vi "Main.vi"() -> ()   [LabVIEW 2017, in "FingerPrintMânager.lvlib"]
doc: "This template is based off of the Queued Message Handler design pattern and the Queued Message Handler project template that ships with LabVIEW.\n\nThe main difference is that the queue is private to this module and communication between modules is performed via Broadcast and Request events.\n\nRequest events are wrapped in public API methods and are handled in the Event Handling Loop (EHL) of this VI. Any module can register for Broadcast events sent by this module. The EHL generates messages based on user interface actions.\n\nThe Message Handling Loop (MHL) processes messages generated by the EHL, or by other messages. The messages are string values, so new messages can be added easily to the Message Cases case structure in the MHL. Each message cluster can also provide an optional value for Message Data, which is a variant that can be converted to whatever message-specific data is required.\n_____\nBased on Delacor QMH Project Template 4.1.0.59."
uses:
  <vilib>/Delacor/Delacor QMH/Libraries/Module Admin_class/Delacor_lib_QMH_Module Admin.lvclass
  Module Data--cluster.ctl
  Stop Argument--cluster.ctl
  <vilib>/Delacor/Delacor QMH/Libraries/Module Admin_class/Delacor_lib_QMH_Module Admin.lvclass/Delacor_lib_QMH_Module Admin.ctl
  Init Argument--cluster.ctl
  Init (Reply Payload)--cluster.ctl
  UnInit Argument--cluster.ctl
  Write Argument--cluster.ctl
  Write (Reply Payload)--cluster.ctl
  Read Argument--cluster.ctl
  Read (Reply Payload)--cluster.ctl
  <vilib>/Utility/miscctls.llb/LVPointTypeDef.ctl
  <vilib>/Delacor/Delacor QMH/Libraries/Module Admin_class/Delacor_lib_QMH_Get External Launch.vi
  <vilib>/Utility/error.llb/Error Cluster From Error Code.vi
  <vilib>/Delacor/Delacor QMH/Libraries/Message Queue_class/Delacor_lib_QMH_Enqueue Message (Single).vi
  <vilib>/ErrorRing/Error Ring.xnode
  <vilib>/Delacor/Delacor QMH/Libraries/Message Queue_class/Delacor_lib_QMH_Message Queue.lvclass
panel:
  out "String":string
  out "VisaRef":refnum<visa-resource-name>
  out "Connected":bool
  in  "Simulate MHL Error":bool
  in  "Simulate EHL Error":bool
  out "error out":errorcluster
  in  "Module Admin":refnum<class "Delacor_lib_QMH_Module Admin.lvclass">
  out "Status":string
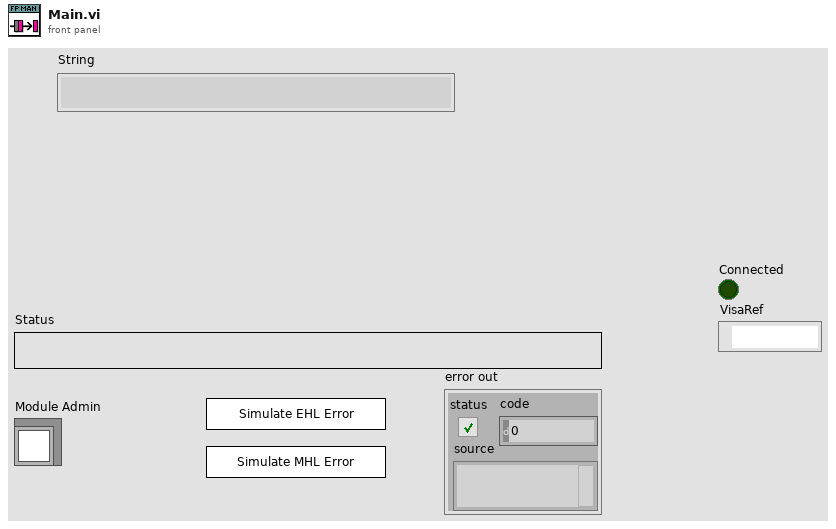
[diagram p1: front panel]
types:
  T1 = typedef "FingerPrintMânager.lvlib/Request Events--cluster.ctl" = cluster{"Stop Module":refnum<user-event>, "Show Panel":refnum<user-event>, "Hide Panel":refnum<user-event>, "Get Module Execution Status":refnum<user-event>, "Show Diagram":refnum<user-event>, "Init":refnum<user-event>, "UnInit":refnum<user-event>, "Write":refnum<user-event>, "Read":refnum<user-event>, "UpdatePump":refnum<user-event>, "StopPump":refnum<user-event>}
  T2 = typedef "FingerPrintMânager.lvlib/Module Data--cluster.ctl" = cluster{"Status":string, "VisaRef":refnum<visa-resource-name>, "Connected":bool}
  T3 = enum32{"invalid lock state", "Not Locked", "Locked (No Password)", "Password-protected"}
  T4 = typedef "FingerPrintMânager.lvlib/Stop Argument--cluster.ctl" = cluster{"Origin":string, "Exit via Stop Module Req?":bool, "Wait for Module to stop?":bool}
  T5 = typedef "FingerPrintMânager.lvlib/Init Argument--cluster.ctl" = cluster{"Wait Notifier":refnum<notifier>, "wait for reply":bool}
  T6 = typedef "FingerPrintMânager.lvlib/UnInit Argument--cluster.ctl" = cluster{"Boolean":bool}
  T7 = typedef "FingerPrintMânager.lvlib/Write Argument--cluster.ctl" = cluster{"Command":string, "Wait Notifier":refnum<notifier>, "wait for reply":bool}
  T8 = typedef "FingerPrintMânager.lvlib/Read Argument--cluster.ctl" = cluster{"Wait Notifier":refnum<notifier>, "wait for reply":bool}
  T9 = typedef "LVPointTypeDef.ctl" = cluster{"Horizontal":i16, "Vertical":i16}
  T10 = enum32{"Invalid", "Standard", "Closed", "Hidden", "Minimized", "Maximized"}
  T11 = typedef "FingerPrintMânager.lvlib/Init (Reply Payload)--cluster.ctl" = cluster{"Connected":bool, "Init_error":errorcluster}
  T12 = typedef "FingerPrintMânager.lvlib/Write (Reply Payload)--cluster.ctl" = cluster{"Status":bool, "Write_error":errorcluster}
  T13 = typedef "FingerPrintMânager.lvlib/Read (Reply Payload)--cluster.ctl" = cluster{"Status":bool, "Response":string, "Read_error":errorcluster}
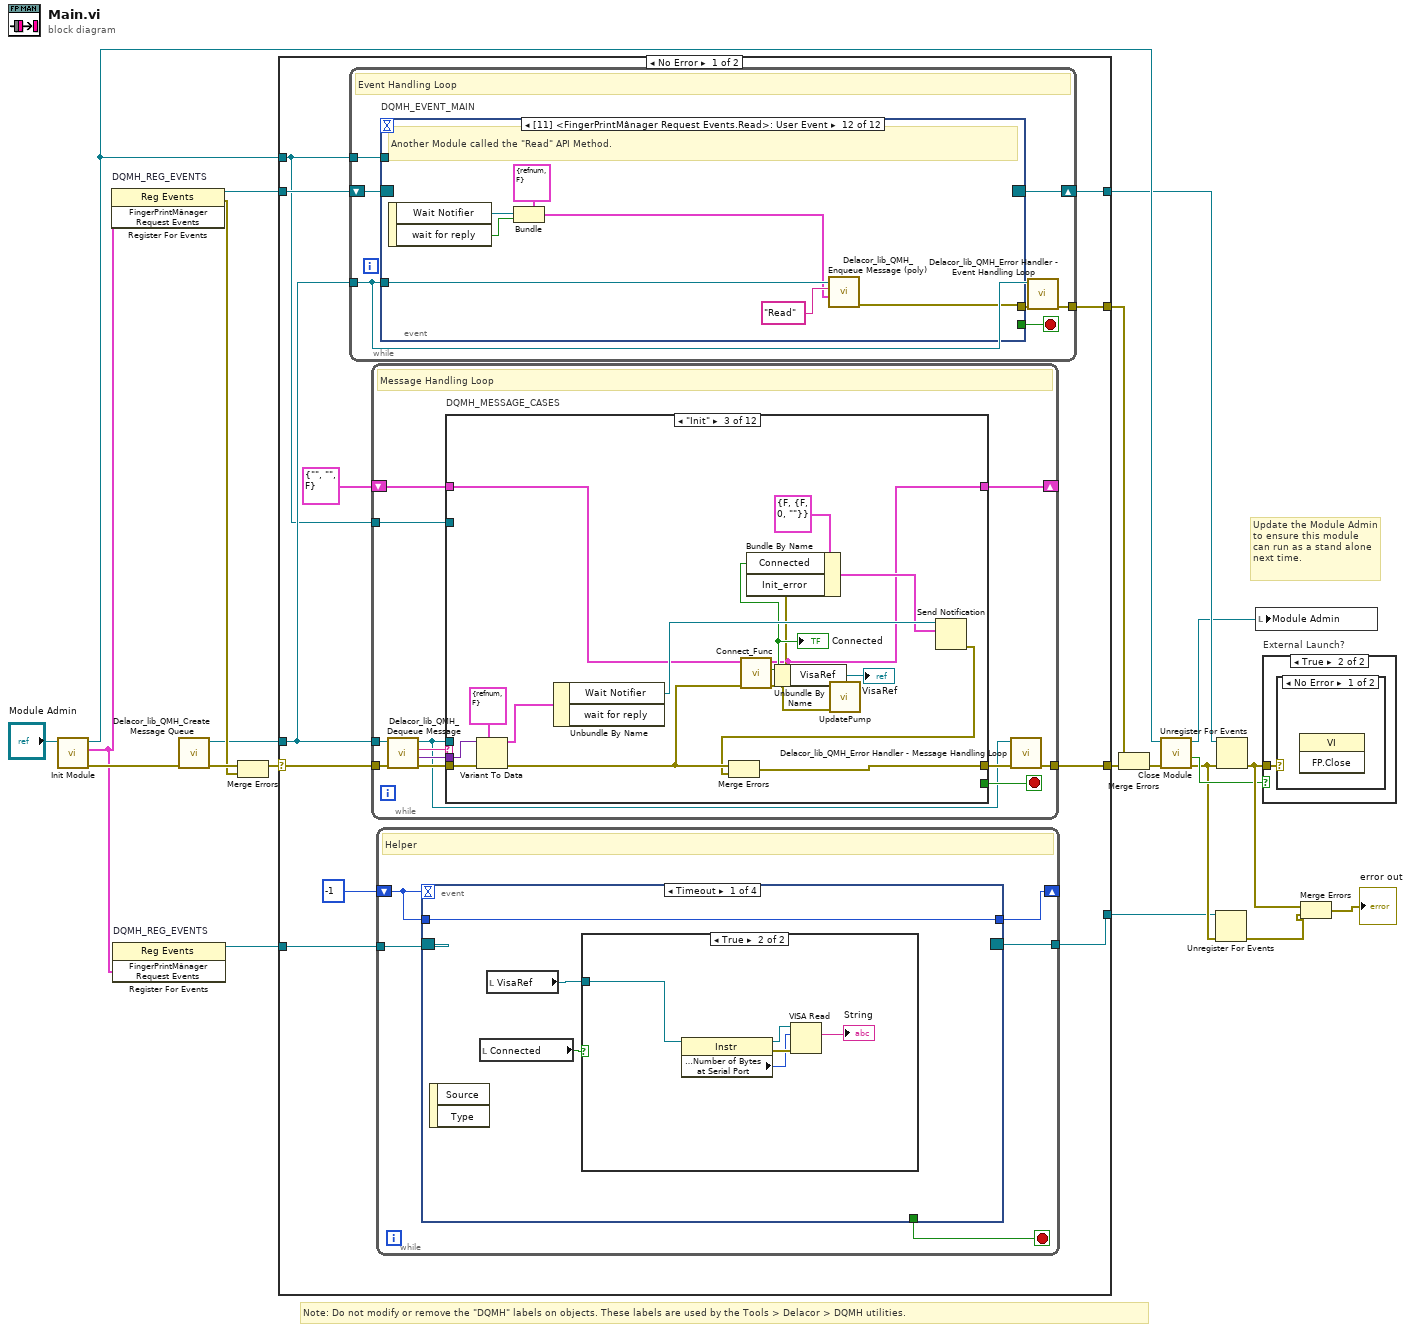
[diagram p0: block diagram]
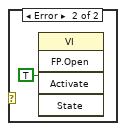
[diagram p3: hidden frame]
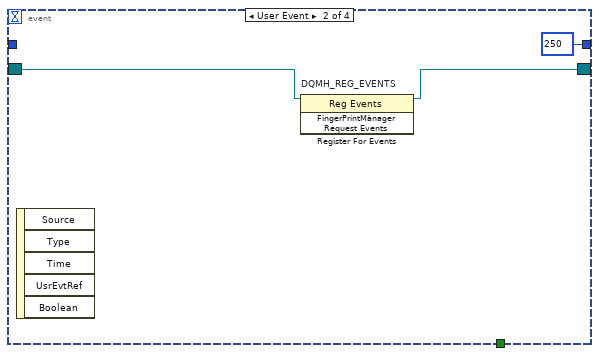
[diagram p5: hidden frame]
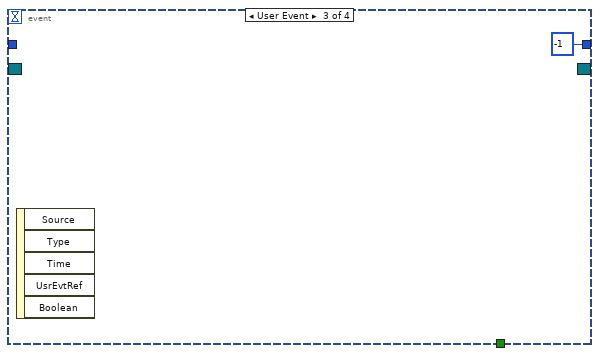
[diagram p6: hidden frame]
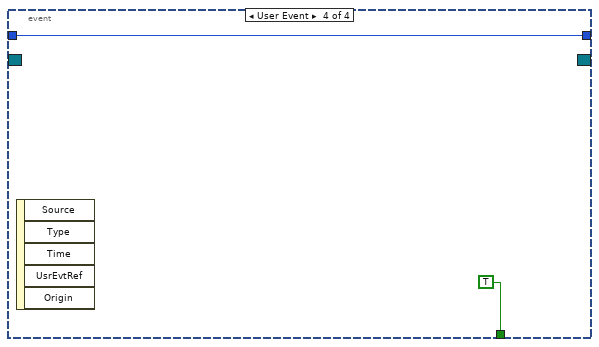
[diagram p7: hidden frame]
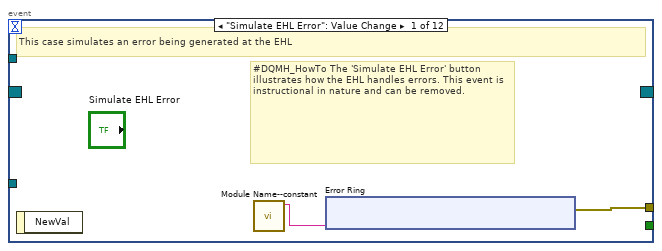
[diagram p8: hidden frame]
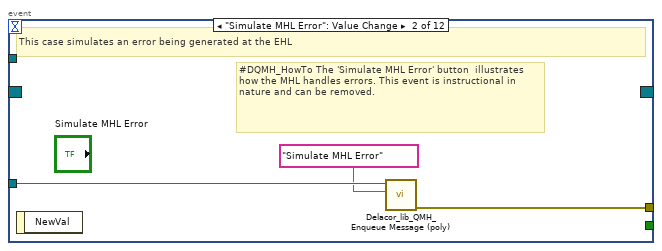
[diagram p9: hidden frame]
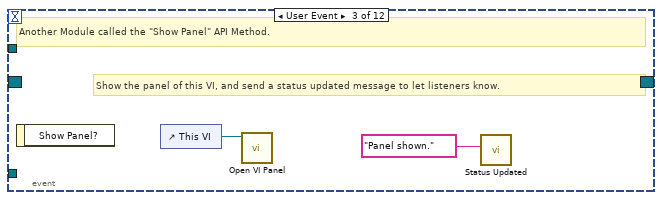
[diagram p10: hidden frame]
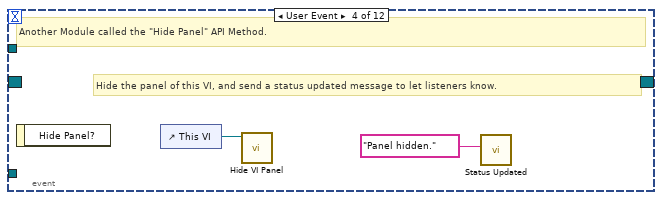
[diagram p11: hidden frame]
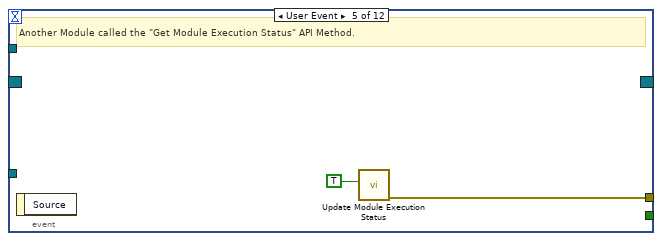
[diagram p12: hidden frame]
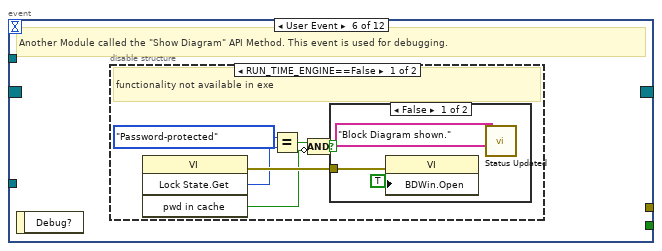
[diagram p13: hidden frame]
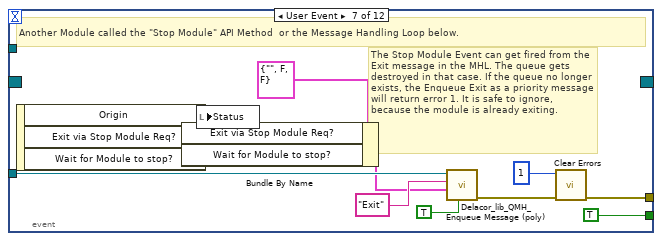
[diagram p16: hidden frame]
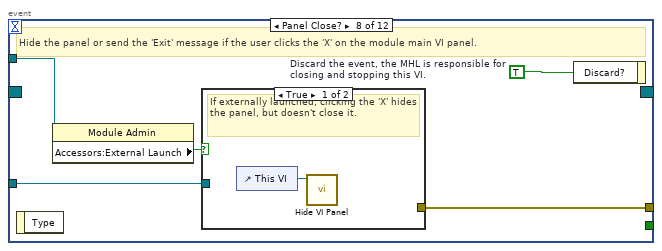
[diagram p17: hidden frame]
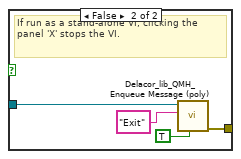
[diagram p18: hidden frame]
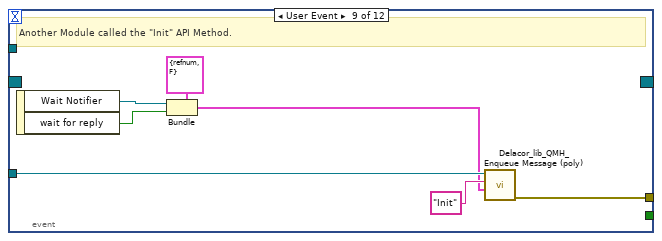
[diagram p19: hidden frame]
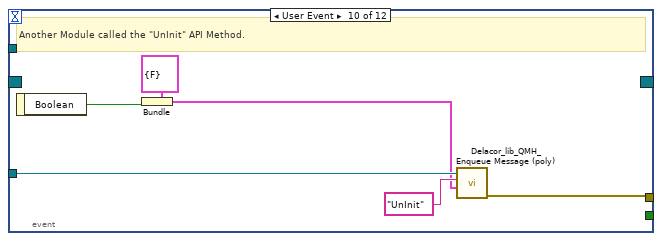
[diagram p20: hidden frame]
diagram:
  # "Note: Do not modify or remove the \"DQMH\" labels on objects. These labels are used by the Tools > Delacor > DQMH utilities."
  # "Update the Module Admin to ensure this module can run as a stand alone next time."
  n1 = call "Init Module.vi"("Singleton Module Admin in"="Module Admin") -> ("error out"=w20:errorcluster, "FingerPrintMânager Request Events"=w6:T1, "Singleton Module Admin out"=w13:refnum<class "Delacor_lib_QMH_Module Admin.lvclass">)  [unwired: 8 in]
  n2 = register-events "DQMH_REG_EVENTS"(w6) -> (reference out=w11:refnum<event-registration>, error out=w14:errorcluster)  [unwired: 2 in]
  n3 = register-events "DQMH_REG_EVENTS"(w6) -> (reference out=w5:refnum<event-registration>)  [unwired: 2 in, 1 out]
  n4 = call <vilib>:"Delacor_lib_QMH_Create Message Queue.vi"("error in (no error)"=w20) -> ("error out"=w16:errorcluster, "Message Queue"=w10:refnum<class "Delacor_lib_QMH_Message Queue.lvclass">)  [unwired: 9 in]
  n5 = Merge Errors(w16, w14) -> (w15:errorcluster)
  n6 = case shown="No Error" w15 {
    selector: w15 -> [w30 w309]
    tunnel: [w32 w309] -> w21
    tunnel: [w29 w306] -> w12
    tunnel: w11 -> [w27 w306]
    tunnel: w10 -> [w26 _]
    tunnel: [w31 _] -> w19
    tunnel: w13 -> [w25 w302]
    tunnel: w5 -> [w24 w301]
    tunnel: [w22 w301] -> w1
    frame No Error {
      n7 = while {
        tunnel: w26 -> [w52]
        shift-right: [w55] -> w29
        shift-left: w27 -> [w56]
        tunnel: [w57] -> w31
        tunnel: w25 -> [w53]
        stop <- w54 stop-if-true
        # "Event Handling Loop"
        n8 = event "DQMH_EVENT_MAIN" shown="[11] <FingerPrintMânager Request Events.Read>: User Event" {
          selector: w56 -> [_ _ _ _ _ _ _ _ _ _ _ _]
          dyn-events: [_ _ _ _ _ _ _ _ _ _ _ _] -> w55
          timeout: _ -> [_ _ _ _ _ _ _ _ _ _ _ _]
          tunnel: [_ _ _ _ _ _ TRUE ("Discard?") _ _ _ _ _] -> w54
          tunnel: w52 -> [_ w69 _ _ _ _ w93 w100 w114 w120 w128 w135]
          tunnel: [w60 w70 _ _ w76 _ w96 w102 w108 w115 w121 w129] -> w58
          tunnel: w53 -> [_ _ _ _ _ _ _ w99 _ _ _ _]
          event "Simulate EHL Error": Value Change {
            # "#DQMH_HowTo The 'Simulate EHL Error' button  illustrates how the EHL handles errors. This event is instructional in nature and can be removed."
            # "This case simulates an error being generated at the EHL"
            n9 = event-data() -> ()  [unwired: 1 in, 1 out]
            n10 = call "Module Name--constant.vi"() -> ("Module Name"=w59:string)  [unwired: 11 in]
            n11 = xnode "Error Ring"("parameter 0"=w59) -> ("error out"=w60:errorcluster)
          }
          event "Simulate MHL Error": Value Change {
            # "#DQMH_HowTo The 'Simulate MHL Error' button  illustrates how the MHL handles errors. This event is instructional in nature and can be removed."
            # "This case simulates an error being generated at the EHL"
            n12 = event-data() -> ()  [unwired: 1 in, 1 out]
            n13 = call-poly <vilib>:"Delacor_lib_QMH_Enqueue Message (poly).vi"("Message"="Simulate MHL Error", "Message Queue in"=w69) -> ("error out"=w70:errorcluster)  [unwired: 8 in, 1 out]
          }
          event User Event {
            # "Show the panel of this VI, and send a status updated message to let listeners know."
            # "Another Module called the \"Show Panel\" API Method."
            n14 = event-data() -> ()  [unwired: 1 in, 1 out]
            n15 = control-ref of="This VI"() -> (w72:refnum<vi>)
            n16 = call "Open VI Panel.vi"("VI"=w72) -> ()  [unwired: 10 in, 1 out]
            n17 = call "Status Updated.vi"("Status"="Panel shown." ("format string")) -> ()  [unwired: 10 in, 1 out]
          }
          event User Event {
            # "Hide the panel of this VI, and send a status updated message to let listeners know."
            # "Another Module called the \"Hide Panel\" API Method."
            n18 = event-data() -> ()  [unwired: 1 in, 1 out]
            n19 = control-ref of="This VI"() -> (w74:refnum<vi>)
            n20 = call "Hide VI Panel.vi"("VI"=w74) -> ()  [unwired: 10 in, 1 out]
            n21 = call "Status Updated.vi"("Status"="Panel hidden." ("format string")) -> ()  [unwired: 10 in, 1 out]
          }
          event User Event {
            # "Another Module called the \"Get Module Execution Status\" API Method."
            n22 = event-data() -> ()  [unwired: 1 in, 1 out]
            n23 = call "Update Module Execution Status.vi"("Running?"=TRUE) -> ("error out"=w76:errorcluster)  [unwired: 10 in]
          }
          event User Event {
            # "Another Module called the \"Show Diagram\" API Method. This event is used for debugging."
            n24 = event-data() -> ()  [unwired: 1 in, 1 out]
            n25 = disable-structure shown="RUN_TIME_ENGINE==False" {
              frame condition #0 (active) {
                # "functionality not available in exe"
                n26 = invoke class="VI" method="Lock State.Get"() -> (error out=w82:errorcluster, "Get Lock State"=w81:T3, "pwd in cache"=w78:bool)  [unwired: 4 in, 1 out]
                n27 = Equal?(x=T3."Password-protected", y=w81) -> (x = y?=w79:bool)
                n28 = Compound Arithmetic op=AND(w79, invert w78) -> (w77:bool)
                n29 = case shown="False" w77 {
                  tunnel: w82 -> [w85 _]
                  frame False {
                    n30 = property class="VI"(error in=w85, "BDWin.Open"=TRUE ("Block Diagram Window:Open")) -> ()  [unwired: 1 in, 2 out]
                    n31 = call "Status Updated.vi"("Status"="Block Diagram shown." ("format string")) -> ()  [unwired: 10 in, 1 out]
                  }
                  frame True {
                    # "Password-protected VI, and the password is not in the cache. Do not show the diagram."
                  }
                }
              }
              frame condition #1 {
              }
            }
          }
          event User Event {
            # "The Stop Module Event can get fired from the Exit message in the MHL. The queue gets destroyed in that case. If the queue no longer exists, the Enqueue Exit as a priority message will return error 1. It is safe to ignore, because the module is already exiting."
            # "Another Module called the \"Stop Module\" API Method  or the Message Handling Loop below."
            n32 = event-data() -> ("Origin"=w92:string, "Exit via Stop Module Req?"=w88:bool, "Wait for Module to stop?"=w87:bool)  [unwired: 1 in]
            n33 = Bundle By Name(cluster=T4 {"Origin"="", "Exit via Stop Module Req?"=FALSE, "Wait for Module to stop?"=FALSE} ("Stop Argument"), "Exit via Stop Module Req?"=w88, "Wait for Module to stop?"=w87) -> (w86:T4)
            n34 = local write "Status"(w92) -> ()
            n35 = call-poly <vilib>:"Delacor_lib_QMH_Enqueue Message (poly).vi"("Priority Message? (F)"=TRUE, "Message Data"=w86, "Message"="Exit", "Message Queue in"=w93) -> ("error out"=w97:errorcluster)  [unwired: 6 in, 1 out]
            n36 = call <vilib>:"Clear Errors.vi"("error in (no error)"=w97, "specific error code to clear (0: all)"=1) -> ("error out"=w96:errorcluster)  [unwired: 4 in, 1 out]
          }
          event Panel Close? {
            w101 = TRUE  # Discard the event, the MHL is responsible for closing and stopping this VI.
            # "Hide the panel or send the 'Exit' message if the user clicks the 'X' on the module main VI panel."
            n37 = event-data() -> ()  [unwired: 1 in, 1 out]
            n38 = property class="Module Admin"(reference=w99) -> ("Accessors:External Launch"=w98:bool)  [unwired: 1 in, 2 out]
            n39 = case shown="True" w98 {
              tunnel: w100 -> [_ w106]
              tunnel: [_ w107] -> w102
              frame True {
                # "If externally launched, clicking the 'X' hides the panel, but doesn't close it."
                n40 = control-ref of="This VI"() -> (w103:refnum<vi>)
                n41 = call "Hide VI Panel.vi"("VI"=w103) -> ()  [unwired: 10 in, 1 out]
              }
              frame False {
                # "If run as a stand-alone VI, clicking the panel 'X' stops the VI."
                n42 = call-poly <vilib>:"Delacor_lib_QMH_Enqueue Message (poly).vi"("Priority Message? (F)"=TRUE, "Message"="Exit", "Message Queue in"=w106) -> ("error out"=w107:errorcluster)  [unwired: 7 in, 1 out]
              }
            }
            n43 = event-data("Discard?"=w101) -> ()  [unwired: 1 in, 1 out]
          }
          event User Event {
            # "Another Module called the \"Init\" API Method."
            n44 = event-data() -> ("Wait Notifier"=w110:refnum<notifier>, "wait for reply"=w109:bool)  [unwired: 1 in]
            n45 = Bundle(cluster=T5 {"Wait Notifier"=refnum, "wait for reply"=FALSE} ("Init Argument"), "Wait Notifier"=w110, "wait for reply"=w109) -> (w111:T5)
            n46 = call-poly <vilib>:"Delacor_lib_QMH_Enqueue Message (poly).vi"("Message Data"=w111, "Message"="Init", "Message Queue in"=w114) -> ("error out"=w108:errorcluster)  [unwired: 7 in, 1 out]
          }
          event User Event {
            # "Another Module called the \"UnInit\" API Method."
            n47 = event-data() -> ("Boolean"=w116:bool)  [unwired: 1 in]
            n48 = Bundle(cluster=T6 {"Boolean"=FALSE} ("UnInit Argument"), "Boolean"=w116) -> (w117:T6)
            n49 = call-poly <vilib>:"Delacor_lib_QMH_Enqueue Message (poly).vi"("Message Data"=w117, "Message"="UnInit", "Message Queue in"=w120) -> ("error out"=w115:errorcluster)  [unwired: 7 in, 1 out]
          }
          event User Event {
            # "Another Module called the \"Write\" API Method."
            n50 = event-data() -> ("Command"=w124:string, "Wait Notifier"=w123:refnum<notifier>, "wait for reply"=w122:bool)  [unwired: 1 in]
            n51 = Bundle(cluster=T7 {"Command"="", "Wait Notifier"=refnum, "wait for reply"=FALSE} ("Write Argument"), "Command"=w124, "Wait Notifier"=w123, "wait for reply"=w122) -> (w125:T7)
            n52 = call-poly <vilib>:"Delacor_lib_QMH_Enqueue Message (poly).vi"("Message Data"=w125, "Message"="Write", "Message Queue in"=w128) -> ("error out"=w121:errorcluster)  [unwired: 7 in, 1 out]
          }
          event User Event {
            # "Another Module called the \"Read\" API Method."
            n53 = event-data() -> ("Wait Notifier"=w131:refnum<notifier>, "wait for reply"=w130:bool)  [unwired: 1 in]
            n54 = Bundle(cluster=T8 {"Wait Notifier"=refnum, "wait for reply"=FALSE} ("Read Argument"), "Wait Notifier"=w131, "wait for reply"=w130) -> (w132:T8)
            n55 = call-poly <vilib>:"Delacor_lib_QMH_Enqueue Message (poly).vi"("Message Data"=w132, "Message"="Read", "Message Queue in"=w135) -> ("error out"=w129:errorcluster)  [unwired: 7 in, 1 out]
          }
        }
        n56 = call-dynamic "Delacor_lib_QMH_Error Handler - Event Handling Loop.vi"("error in (no error)"=w58, "Message Queue in"=w52) -> ("dup error in"=w57:errorcluster)  [unwired: 8 in, 1 out]
      }
      n57 = while {
        tunnel: w26 -> [w138]
        shift-right: [w142] -> _
        shift-left: T2 {"Status"="", "VisaRef"="", "Connected"=FALSE} ("Data Cluster") -> [w143]
        tunnel: w30 -> [w146]
        tunnel: [w144] -> w32
        tunnel: w25 -> [w136]
        stop <- w141 stop-if-true
        # "Message Handling Loop"
        n58 = call-dynamic "Delacor_lib_QMH_Dequeue Message.vi"("error in (no error)"=w146, "Message Queue in"=w138) -> ("error out"=w145:errorcluster, "Message Data"=w139:variant, "Message"=w140:string, "Message Queue out"=w137:refnum<class "Delacor_lib_QMH_Message Queue.lvclass">)  [unwired: 6 in]
        n59 = case "DQMH_MESSAGE_CASES" shown="\"Init\"" w140 {
          selector: w140 -> [_ _ _ _ _ _ _ _ _ _ _ w288]
          tunnel: w137 -> [_ _ _ _ _ _ _ _ _ w258 w280 _]
          tunnel: w145 -> [w165 w169 w184 w196 w220 w238 w241 w243 w248 w265 w286 w290]
          tunnel: [w163 w169 w177 w189 w213 w231 w240 w243 w247 w261 w283 w291] -> w147
          tunnel: w143 -> [w154 w168 w176 w192 w212 w230 w239 w242 w245 w260 w279 w289]
          tunnel: [w153 w168 w171 w186 w210 w229 w239 w242 w245 w260 w279 w289] -> w142
          tunnel: [_ _ _ _ _ _ _ _ _ _ w278 _] -> w141
          tunnel: w139 -> [_ _ w183 w195 w219 w237 _ _ _ w259 w277 _]
          tunnel: w136 -> [w155 _ _ _ _ _ _ _ _ w257 w272 _]
          frame "Initialize" {
            w148 = "Initial Message" ("Initial Message")
            # "#CodeNeeded - Initialize the appearance of the front panel."
            # "#CodeNeeded - Initialize your state data here."
            # "Initialize - Any operation that needs to be done before the module can receive messages. Synchronize Caller Events.vi will inform Start Module.vi that the module has launched and is ready to receive messages. Module Did Init.vi will broadcast that the module initialized."
            n60 = call "Synchronize Caller Events.vi"("error in (no error)"=w165, "Singleton Module Admin in"=w155) -> ("error out"=w164:errorcluster, "Singleton Module Admin out"=w150:refnum<class "Delacor_lib_QMH_Module Admin.lvclass">)  [unwired: 8 in]
            n61 = property class="Module Admin"(reference=w150) -> ("Accessors:External Launch"=w159:bool)  [unwired: 1 in, 2 out]
            n62 = Select(t=T10."Hidden" ("State"), s=w159, f=T10."Standard" ("State")) -> (s? t:f=w156:T10)
            n63 = call "Module Name--constant.vi"() -> ("Module Name"=w162:string)  [unwired: 11 in]
            n64 = property class="VI"("Front Panel.Title"=w162) -> (reference out=w161:refnum<vi>, error out=w167:errorcluster)  [unwired: 2 in]
            n65 = call "Module Name--constant.vi"() -> ("Module Name"=w151:string)  [unwired: 11 in]
            n66 = invoke class="VI" method="FP.Open"(reference=w161, error in=w167, "State"=w156) -> (reference out=w160:refnum<vi>, error out=w166:errorcluster)  [unwired: 2 in, 3 out]
            n67 = Bundle By Name(cluster=w154, "Status"=w148) -> (w153:T2)
            n68 = call "Module Did Init.vi"("error in (no error)"=w164, "Initialized?"=TRUE, "Origin"=w151) -> ("error out"=w163:errorcluster)  [unwired: 8 in]
            n69 = invoke class="VI" method="FP.Center"(reference=w160, error in=w166) -> ()  [unwired: 1 in, 3 out]
            n70 = property on="Pane" class="Pane"("Origin"=T9 {"Horizontal"=0, "Vertical"=0}) -> ()  [unwired: 2 in, 2 out]
            "Status" <- w148
          }
          frame "--- Module Specific ---" {
            # "Separator -- The following cases handle messages specific to this Module."
          }
          frame "Init" {
            n71 = Variant To Data(error in=w184, type=T5 {"Wait Notifier"=refnum, "wait for reply"=FALSE} ("Init Argument"), Variant=w183) -> (data=w181:T5, error out=w175:errorcluster)
            n72 = Unbundle By Name(w181) -> ("Wait Notifier"=w180:refnum<notifier>)  [unwired: 1 out]
            n73 = call "Connect_Func.vi"("error in (no error)"=w175, "Data Cluster in"=w176) -> ("error out"=w172:errorcluster, "Connected"=w173:bool, "Data Cluster out"=w171:T2)  [unwired: 7 in]
            "Connected" <- w173
            n74 = Bundle By Name(cluster=T11 {"Connected"=FALSE, "Init_error"={"status"=FALSE, "code"=0, "source"=""}} ("Init (Reply Payload)"), "Connected"=w173, "Init_error"=w172) -> (w179:T11)
            n75 = Unbundle By Name(w171) -> ("VisaRef"=→"VisaRef":refnum<visa-resource-name>)
            n76 = call "UpdatePump.vi"("error in (no error)"=w172) -> ()  [unwired: 10 in, 1 out]
            n77 = Send Notification(notification=w179, notifier=w180) -> (error out=w174:errorcluster)  [unwired: 1 in, 1 out]
            n78 = Merge Errors(w175, w174) -> (w177:errorcluster)
          }
          frame "UnInit" {
            n79 = Variant To Data(error in=w196, type=T6 {"Boolean"=FALSE} ("UnInit Argument"), Variant=w195) -> (data=w193:T6, error out=w188:errorcluster)
            n80 = Unbundle By Name(w192) -> ("VisaRef"=w190:refnum<visa-resource-name>, "Connected"=w191:bool)
            n81 = Unbundle By Name(w193) -> ()  [unwired: 1 out]
            n82 = case shown="True" w191 {
              selector: w191 -> [w197 _]
              tunnel: w190 -> [_ w202]
              tunnel: w188 -> [w198 w201]
              tunnel: [w198 w200] -> w187
              tunnel: [w197 FALSE] -> w185
              frame False {
              }
              frame True {
                n83 = VISA Close(VISA resource name=w202, error in (no error)=w201) -> (error out=w200:errorcluster)
              }
            }
            n84 = Bundle By Name(cluster=w192, "Connected"=w185) -> (w186:T2)
            n85 = call <vilib>:"Clear Errors.vi"("error in (no error)"=w187) -> ("error out"=w189:errorcluster)  [unwired: 5 in, 1 out]
          }
          frame "Write" {
            n86 = Variant To Data(error in=w220, type=T7 {"Command"="", "Wait Notifier"=refnum, "wait for reply"=FALSE} ("Write Argument"), Variant=w219) -> (data=w217:T7, error out=w208:errorcluster)
            n87 = Unbundle By Name(w212) -> ("VisaRef"=w211:refnum<visa-resource-name>)
            n88 = Unbundle By Name(w217) -> ("Command"=w207:string, "Wait Notifier"=w216:refnum<notifier>)  [unwired: 1 out]
            n89 = VISA Write(VISA resource name=w211, write buffer=w207, error in (no error)=w208) -> (VISA resource name out=w209:refnum<visa-resource-name>, error out=w206:errorcluster)  [unwired: 1 out]
            n90 = case shown="No Error" w206 {
              selector: w206 -> [w221 w223]
              tunnel: [TRUE _] -> w205
              tunnel: [w221 w223] -> w204
              frame No Error {
              }
              frame Error {
              }
            }
            n91 = Bundle By Name(cluster=T12 {"Status"=FALSE, "Write_error"={"status"=FALSE, "code"=0, "source"=""}} ("Write (Reply Payload)"), "Status"=w205, "Write_error"=w204) -> (w215:T12)
            n92 = Bundle By Name(cluster=w212, "VisaRef"=w209) -> (w210:T2)
            n93 = Send Notification(notification=w215, notifier=w216) -> (error out=w203:errorcluster)  [unwired: 1 in, 1 out]
            n94 = Merge Errors(w208, w203) -> (w213:errorcluster)
          }
          frame "Read" {
            n95 = Variant To Data(error in=w238, type=T8 {"Wait Notifier"=refnum, "wait for reply"=FALSE} ("Read Argument"), Variant=w237) -> (data=w235:T8, error out=w228:errorcluster)
            n96 = Unbundle By Name(w235) -> ("Wait Notifier"=w234:refnum<notifier>)  [unwired: 1 out]
            n97 = call "Read_func.vi"("error in (no error)"=w228, "Data Cluster in"=w230) -> ("error out"=w227:errorcluster, "read buffer"=w226:string, "Data Cluster out"=w229:T2, "Status"=w225:bool)  [unwired: 5 in, 1 out]
            n98 = Bundle By Name(cluster=T13 {"Status"=FALSE, "Response"="", "Read_error"={"status"=FALSE, "code"=0, "source"=""}} ("Read (Reply Payload)"), "Status"=w225, "Response"=w226, "Read_error"=w227) -> (w233:T13)
            n99 = Send Notification(notification=w233, notifier=w234) -> (error out=w224:errorcluster)  [unwired: 1 in, 1 out]
            n100 = Merge Errors(w228, w224) -> (w231:errorcluster)
          }
          frame "---Copy This Frame---" {
            # "Duplicate this frame when creating new messages.  Change this comment in the duplicated frame to describe this message."
            n101 = Merge Errors(w241) -> (w240:errorcluster)
          }
          frame "--- Exit and Error Handling---" {
            # "Separator - The following cases handle errors and exit messages."
          }
          frame "Simulate MHL Error" {
            # "#DQMH_HowTo The 'Simulate MHL Error' button  illustrates how the MHL handles errors. This event is instructional in nature and can be removed."
            # "Simulate an error occurring at the MHL"
            n102 = call "Module Name--constant.vi"() -> ("Module Name"=w244:string)  [unwired: 11 in]
            n103 = xnode "Error Ring"("parameter 0"=w244) -> ("error out"=w246:errorcluster)
            n104 = Merge Errors(w248, w246) -> (w247:errorcluster)
          }
          frame "Error" {
            # "#CodeRecommended - If you ever change the name of this \"Error\" message, you'll need to update the name in the Check Loop Error.vi as well."
            # "#CodeRecommended - If the module is running in standalone mode (External Launch = FALSE), this code will pop up an error dialog and call the 'Exit' message if an error occurs. Add more fine-grained error handling here."
            # "Error - Check the error message data and respond accordingly. This message is sent by the \"Error Handler\" VIs at the end of each loop in this application."
            n105 = property class="Module Admin"(reference=w257) -> ("Accessors:External Launch"=w256:bool)  [unwired: 1 in, 2 out]
            n106 = Variant To Data(error in=w265, type=errorcluster {"status"=FALSE, "code"=0, "source"=""} ("error constant"), Variant=w259) -> (data=w266:errorcluster, error out=w263:errorcluster)
            n107 = call "Error Reported.vi"("Error"=w266) -> ()  [unwired: 10 in, 1 out]
            n108 = case shown="False" w256 {
              tunnel: [w271 _] -> w262
              tunnel: w258 -> [w269 _]
              tunnel: w266 -> [w270 _]
              frame False {
                # "If the module is running standalone, then pop up an error dialog and call the \"Exit\" message."
                n109 = call <vilib>:"Simple Error Handler.vi"("error in (no error)"=w270) -> ()  [unwired: 4 in, 5 out]
                n110 = call-poly <vilib>:"Delacor_lib_QMH_Enqueue Message (poly).vi"("Priority Message? (F)"=TRUE, "Message"="Exit", "Message Queue in"=w269) -> ("error out"=w271:errorcluster)  [unwired: 7 in, 1 out]
              }
              frame True {
                # "If the module was launched externally, calling the Error Reported broadcast VI is the only action performed by the \"Error\" message. The module's caller can then process the error appropriately."
              }
            }
            n111 = Merge Errors(w263, w262) -> (w261:errorcluster)
            n112 = local write "error out"(w261) -> ()
          }
          frame "Exit" {
            w276 = 91  # 91: not all Exit messages will have an argument
            w278 = TRUE  # Stop the VI
            # "Release the message queue reference"
            # "#CodeNeeded - Add any required cleanup code here"
            # "Exit - Exit the application."
            n113 = Variant To Data(error in=w286, type=T4 {"Origin"="", "Exit via Stop Module Req?"=FALSE, "Wait for Module to stop?"=FALSE} ("Stop Argument"), Variant=w277) -> (data=w274:T4, error out=w282:errorcluster)
            n114 = call <vilib>:"Clear Errors.vi"("error in (no error)"=w282, "specific error code to clear (0: all)"=w276) -> ("error out"=w285:errorcluster)  [unwired: 4 in, 1 out]
            n115 = control-ref of="This VI"() -> (w273:refnum<vi>)
            n116 = call-dynamic "Delacor_lib_QMH_Release Message Queue.vi"("error in (no error)"=w285, "Message Queue"=w280) -> ("error out"=w284:errorcluster)  [unwired: 9 in]
            n117 = call "Handle Exit.vi"("Stop Argument"=w274, "Admin in"=w272, "VI reference"=w273) -> ("error out"=w281:errorcluster)  [unwired: 7 in, 1 out]
            n118 = Merge Errors(w284, w281) -> (w283:errorcluster)
          }
          frame Default {
            # "'Default' case only runs if there is a message that isn't defined in any of the other cases.  Output a programming error."
            n119 = call "Module Name--constant.vi"() -> ("Module Name"=w287:string)  [unwired: 11 in]
            n120 = xnode "Error Ring"("parameter 0"=w288, "parameter 1"=w287) -> ("error out"=w292:errorcluster)
            n121 = Merge Errors(w290, w292) -> (w291:errorcluster)
          }
        }
        n122 = call-dynamic "Delacor_lib_QMH_Error Handler - Message Handling Loop.vi"("error in (no error)"=w147, "Message Queue in"=w137) -> ("dup error in"=w144:errorcluster)  [unwired: 8 in, 1 out]
      }
      n123 = while {
        tunnel: w24 -> [w37]
        shift-right: [w35] -> _
        shift-left: -1 -> [w34]
        tunnel: [w33] -> w22
        stop <- w36 stop-if-true
        # "Helper"
        n124 = event shown="[0] Timeout" {
          selector: w37 -> [_ w48 _ _]
          dyn-events: [_ w47 _ _] -> w33
          timeout: w34 -> [_ _ _ _]
          tunnel: [_ _ _ TRUE] -> w36
          tunnel: [w40 250 -1 w50] -> w35
          tunnel: w34 -> [w40 _ _ w50]
          event Timeout {
            n125 = event-data() -> ()  [unwired: 1 in, 2 out]
            n126 = local read "Connected"() -> (w39:bool)
            n127 = local read "VisaRef"() -> (w38:refnum<visa-resource-name>)
            n128 = case shown="True" w39 {
              tunnel: w38 -> [_ w42]
              frame False {
              }
              frame True {
                n129 = property class="Instr"(reference=w42) -> (reference out=w45:refnum<visa-resource-name>, error out=w44:errorcluster, "Serial Settings:Number of Bytes at Serial Port"=w43:u32)  [unwired: 1 in]
                n130 = VISA Read(VISA resource name=w45, byte count=w43, error in (no error)=w44) -> (read buffer=→"String":string)  [unwired: 3 out]
              }
            }
          }
          event User Event {
            n131 = event-data() -> ()  [unwired: 1 in, 5 out]
            n132 = register-events "DQMH_REG_EVENTS"(reference=w48) -> (reference out=w47:refnum<event-registration>)  [unwired: 2 in, 1 out]
          }
          event User Event {
            n133 = event-data() -> ()  [unwired: 1 in, 5 out]
          }
          event User Event {
            n134 = event-data() -> ()  [unwired: 1 in, 5 out]
          }
        }
      }
    }
    frame Error {
      # "Synchronize Caller Events.vi will inform Start Module.vi that the module has launched and will let the code calling Start Module.vi register for broadcasts and would permit the caller receive the broadcast that an error occurred at launch time."
      n135 = call "Synchronize Caller Events.vi"("Singleton Module Admin in"=w302) -> ("error out"=w307:errorcluster)  [unwired: 9 in, 1 out]
      n136 = call "Module Name--constant.vi"() -> ("Module Name"=w305:string)  [unwired: 11 in]
      n137 = Format Into String(format string="An error occurred during initialization. %s is no longer running.", w305) -> (resulting string=w303:string)  [unwired: 2 in, 1 out]
      n138 = Merge Errors(w309, w307) -> (w308:errorcluster)
      n139 = call "Error Reported.vi"("Additional Information"=w303, "Error"=w308) -> ()  [unwired: 9 in, 1 out]
    }
  }
  n140 = Merge Errors(w19, w21) -> (w18:errorcluster)
  n141 = call "Close Module.vi"("error in (no error)"=w18, "Module Admin in"=w13) -> ("error out"=w2:errorcluster, "External Launch"=w7:bool, "Module Admin out"=w8:refnum<class "Delacor_lib_QMH_Module Admin.lvclass">)  [unwired: 7 in]
  n142 = Unregister For Events(event registration refnum=w1, error in=w2) -> (error out=w3:errorcluster)
  n143 = Unregister For Events(event registration refnum=w12, error in=w2) -> (error out=w17:errorcluster)
  n144 = local write "Module Admin"(w8) -> ()
  n145 = case "External Launch?" shown="True" w7 {
    tunnel: w17 -> [_ w310]
    frame False {
    }
    frame True {
      n146 = case shown="No Error" w310 {
        frame No Error {
          n147 = invoke class="VI" method="FP.Close"() -> ()  [unwired: 3 in, 3 out]
        }
        frame Error {
          n148 = invoke class="VI" method="FP.Open"("Activate"=TRUE ("Activate?")) -> ()  [unwired: 4 in, 5 out]
        }
      }
    }
  }
  n149 = Merge Errors(w17, w3) -> (→"error out":errorcluster)
